vi "Configure Channel.vi"(0 "VISA resource name":refnum<visa-resource-name>, 5 "Channel (1: Channel 1)":u16(ring)=1 items=["Channel 1"=1, "Channel 2"=2, "Channel 3"=3, "Channel 4"=4], 9 "Probe Attenuation (1X)":dbl=1.0 format="%#.0f", 11 "error in (no error)":errorcluster, 12 "Vertical Range (1.0 V)":dbl=1.0, 13 "Vertical Offset (0.0 V)":dbl) -> (4 "VISA resource name out":refnum<visa-resource-name>, 15 "error out":errorcluster)   [LabVIEW 2021, in "Siglent SDS 1000 2000 Series.lvlib"]
doc: "Configures the common properties of the oscilloscope's vertical subsystem for the specified channel. Call this VI for each channel you want to enable to acquire waveforms.\n\nCaveats:\n1. The oscilloscope will not accept a value for Probe Attenuation if there is a probe attached that employs a fixed value for attenuation.\n2. Allowed coupling values depend on what kind of probe is attached, if any.\n\nNote:\nThe channel settings will not be applied if the channel is not enabled."
uses:
  <instrlib>/Siglent SDS 1000 2000 Series/Siglent SDS 1000 2000 Series.lvlib
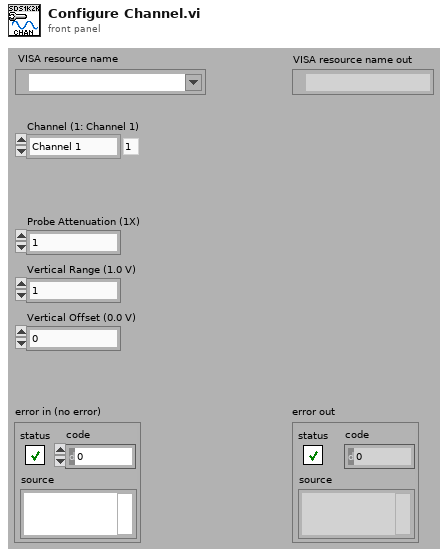
[diagram p1: front panel]
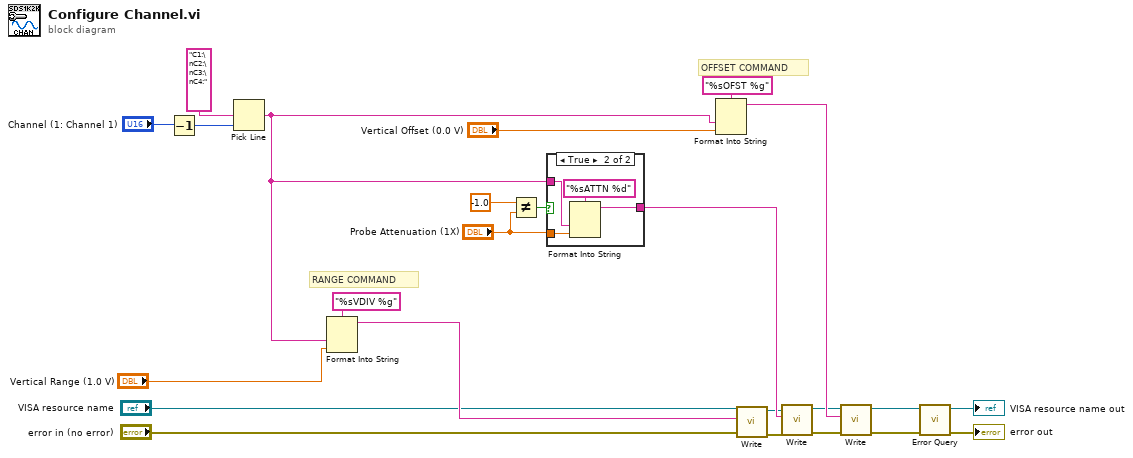
[diagram p0: block diagram]
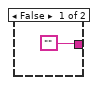
[diagram p2: hidden frame]
diagram:
  # "RANGE COMMAND"
  # "OFFSET COMMAND"
  n1 = Decrement(x="Channel (1: Channel 1)") -> (x-1=w4:u16)
  n2 = Pick Line(multi-line string="C1:\nC2:\nC3:\nC4:", line index=w4) -> (output string=w3:string)  [unwired: 1 in]
  n3 = Format Into String(format string="%sVDIV %g", w3, "Vertical Range (1.0 V)") -> (resulting string=w10:string)  [unwired: 2 in, 1 out]
  n4 = Not Equal?(x=-1.0, y="Probe Attenuation (1X)") -> (x != y?=w16:bool)
  n5 = case shown="True" w16 {
    tunnel: w3 -> [_ w28]
    tunnel: "Probe Attenuation (1X)" -> [_ w27]
    tunnel: ["" ("Empty String Constant") w26] -> w11
    frame False {
    }
    frame True {
      n6 = Format Into String(format string="%sATTN %d" ("Attenuation Command"), w28, w27) -> (resulting string=w26:string)  [unwired: 2 in, 1 out]
    }
  }
  n7 = Format Into String(format string="%sOFST %g", w3, "Vertical Offset (0.0 V)") -> (resulting string=w14:string)  [unwired: 2 in, 1 out]
  n8 = call <instrlib>:"Write.vi"("error in (no error)"="error in (no error)", "Write Buffer"=w10, "VISA resource name"="VISA resource name") -> ("error out"=w8:errorcluster, "VISA resource name out"=w9:refnum<visa-resource-name>)  [unwired: 6 in, 1 out]
  n9 = call <instrlib>:"Write.vi"("error in (no error)"=w8, "Write Buffer"=w11, "VISA resource name"=w9) -> ("error out"=w12:errorcluster, "VISA resource name out"=w13:refnum<visa-resource-name>)  [unwired: 6 in, 1 out]
  n10 = call <instrlib>:"Write.vi"("error in (no error)"=w12, "Write Buffer"=w14, "VISA resource name"=w13) -> ("error out"=w21:errorcluster, "VISA resource name out"=w22:refnum<visa-resource-name>)  [unwired: 6 in, 1 out]
  n11 = call <instrlib>:"Error Query.vi"("error in (no error)"=w21, "VISA resource name"=w22) -> ("error out"=→"error out":errorcluster, "VISA resource name out"=→"VISA resource name out":refnum<visa-resource-name>)  [unwired: 6 in, 2 out]
